vi "array contains cluster with array.vi"() -> ()   [LabVIEW 2017]
uses:
  9f1c8977-aa41-4596-a18a-6dba2ebc59d2.vi
  0333efe5-f0fb-4901-b6dd-db031cec30c6.vi
  API-String-Arugments-Support/_Support/Data To API String Arguments.vi
  API-String-Arugments-Support/_Support/Convert API String Arguments to Data(variant).vi
  <userlib>/_NEVSTOP/Communicable State Machine(CSM)/Communicable State Machine.lvlib
panel:
  out "Array of Strings 2":string[](array[string])=["sin(x)+2", "VIA(x", "y)", " VIB(z)"]
  out "Array of Strings":string[](array[string])=["sin(x)+2", "VIA(x", "y)", " VIB(z)"]
  out "String out":string
  in  "Array":cluster{"String":string, "BoolArray":bool[]}[](array[cluster])=[{"String"="abc", "BoolArray"=[TRUE, FALSE, TRUE, FALSE]}, {"String"="def", "BoolArray"=[FALSE, TRUE, FALSE, TRUE]}, {"String"="xyz", "BoolArray"=[TRUE, TRUE, FALSE, FALSE]}]
  out "Array":cluster{"String":string, "BoolArray":bool[]}[](array[cluster])=[{"String"="abc", "BoolArray"=[TRUE, FALSE, TRUE, FALSE]}, {"String"="def", "BoolArray"=[FALSE, TRUE, FALSE, TRUE]}, {"String"="xyz", "BoolArray"=[TRUE, TRUE, FALSE, FALSE]}]
  out "String":string
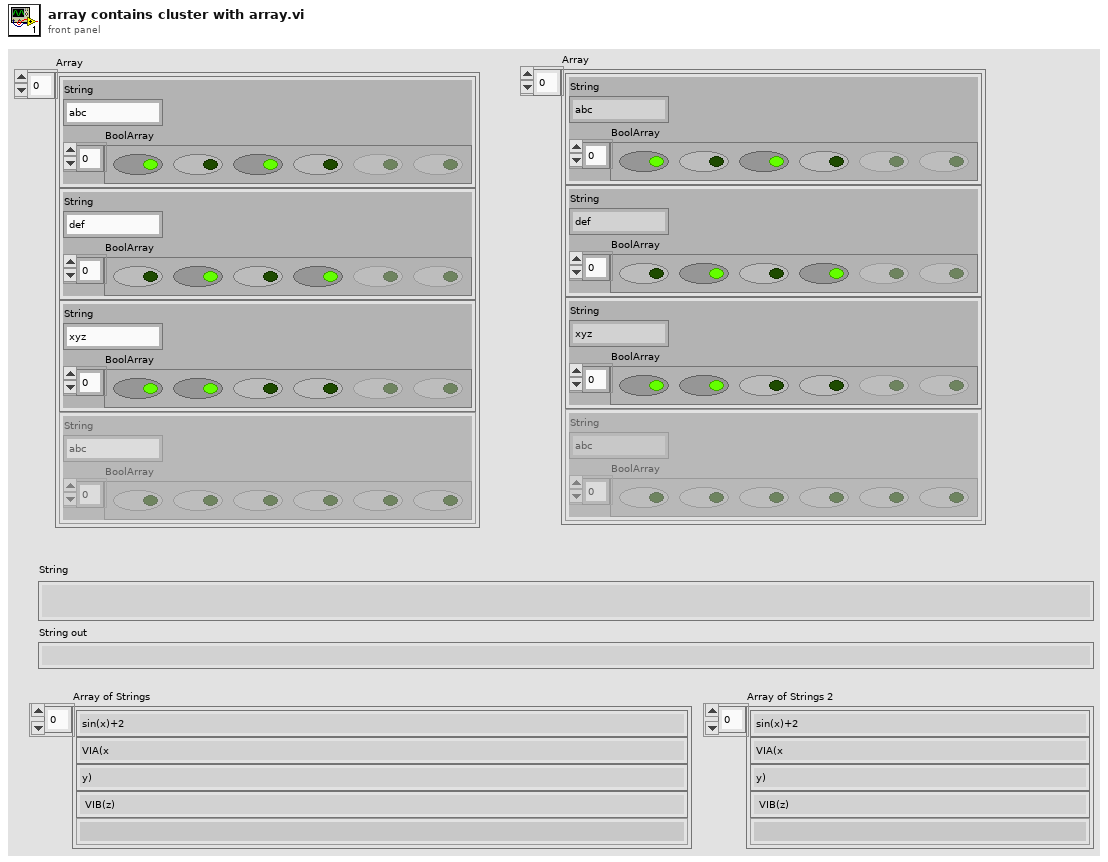
[diagram p1: front panel]
types:
  T1 = enum16{"0x2829 - ()", "0x5B5D - []", "0x7B7D - {}"}
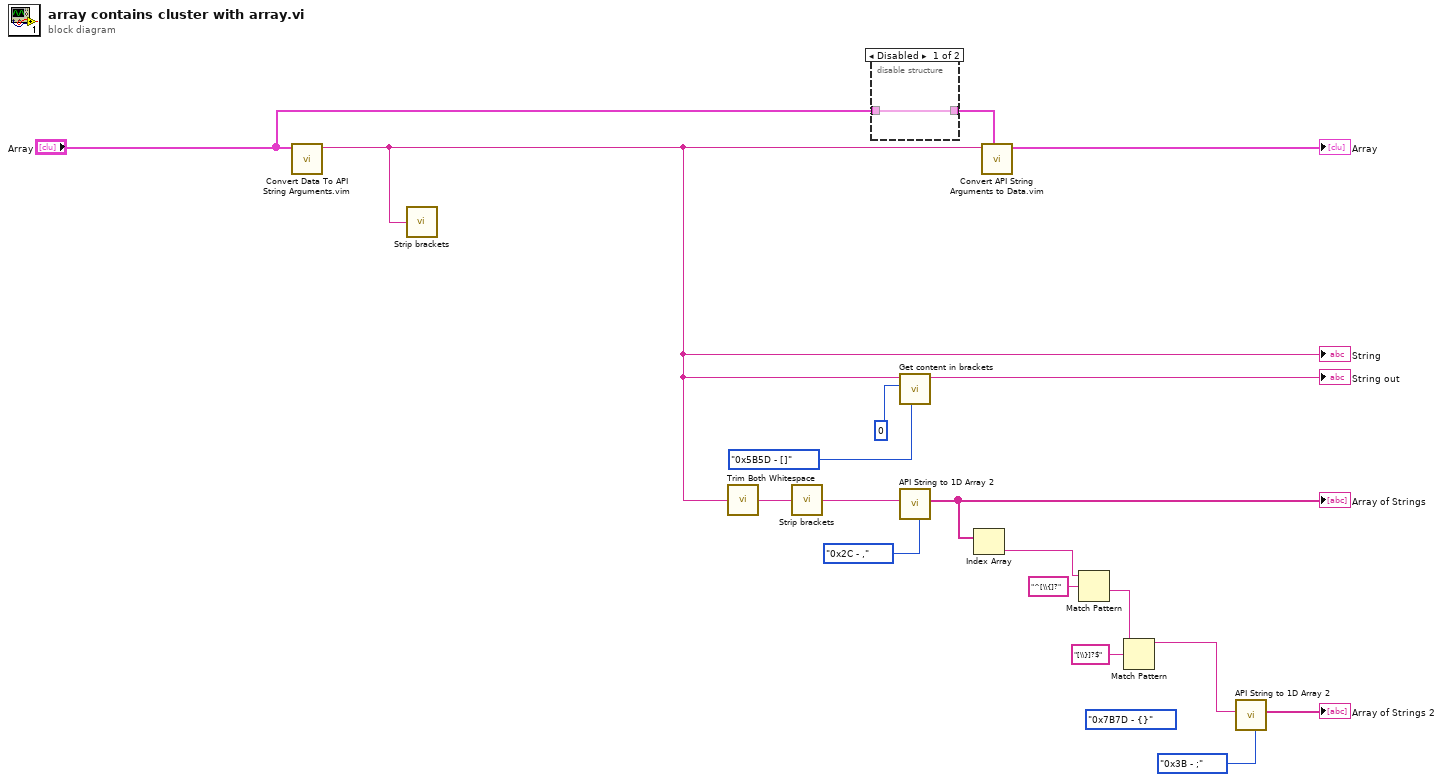
[diagram p0: block diagram]
diagram:
  (unwired) T1."0x7B7D - {}" ("TYPE")
  n1 = call "Convert Data To API String Arguments.vim"("data"="Array") -> ("String"=w4:string)  [unwired: 7 in, 1 out]
  "String" <- w4
  n2 = call "Strip brackets.vi"("trimmed string in"=w4) -> ()  [unwired: 3 in, 1 out]
  n3 = call <userlib>:"Trim Both Whitespace.vi"("string"=w4) -> ("trimmed string"=w5:string)  [unwired: 1 in]
  n4 = call "Strip brackets.vi"("trimmed string in"=w5) -> ("trimmed string out"=w13:string)  [unwired: 3 in]
  n5 = disable-structure "Diagram Disable Structure" shown="Disabled" {
    disable-tunnel: "Array" -> [w19 _]
    disable-tunnel: [w19 _] -> w17
    frame Disabled {
    }
    frame Enabled {
    }
  }
  n6 = call "Get content in brackets.vi"("TYPE"=T1."0x5B5D - []" ("Enum"), "start"=0, "String in"=w4) -> ("String out"=→"String out":string)  [unwired: 7 in, 1 out]
  n7 = call "API String to 1D Array 2.vi"("SEPERATOR"=enum16{"0x2C - ,", "0x3B - ;"}."0x2C - ,", "string"=w13) -> ("Array of Strings"=w12:string[])  [unwired: 8 in, 1 out]
  "Array of Strings" <- w12
  n8 = Index Array(array=w12) -> (element=w8:string)  [unwired: 1 in]
  n9 = call "Convert API String Arguments to Data.vim"("Type"=w17, "String"=w4) -> ("Data"=→"Array":cluster{"String":string, "BoolArray":bool[]}[])  [unwired: 6 in, 1 out]
  n10 = Match Pattern(string=w8, regular expression="^[\\{]?") -> (after substring=w11:string)  [unwired: 1 in, 3 out]
  n11 = Match Pattern(string=w11, regular expression="[\\}]?$") -> (before substring=w7:string)  [unwired: 1 in, 3 out]
  n12 = call "API String to 1D Array 2.vi"("SEPERATOR"=enum16{"0x2C - ,", "0x3B - ;"}."0x3B - ;", "string"=w7) -> ("Array of Strings"=→"Array of Strings 2":string[])  [unwired: 8 in, 1 out]
